vi "Read Enable and Power On Sensor Opcode_MI.vi"(8 "error in (no error)":errorcluster, 10 "Sensor name":string, 11 "MachineInterfaceRecipeOpcodes":T1) -> (0 "error out":errorcluster, 3 "Enable and Power On Sensor Opcodes":string[](array[string]))   [LabVIEW 2019, in "Machine Interface.lvclass"]
uses:
  Machine Interface.lvclass
  Controls/Machine Interface Config File Structure_MI.ctl
panel:
  out "variant":variant
  out "Error Message":string
  out "basePath in":string="$.MachineInterfaceRecipeOpcodes.TriggerLightCameraSequence[Name="
  out "output array":string[](array[string])
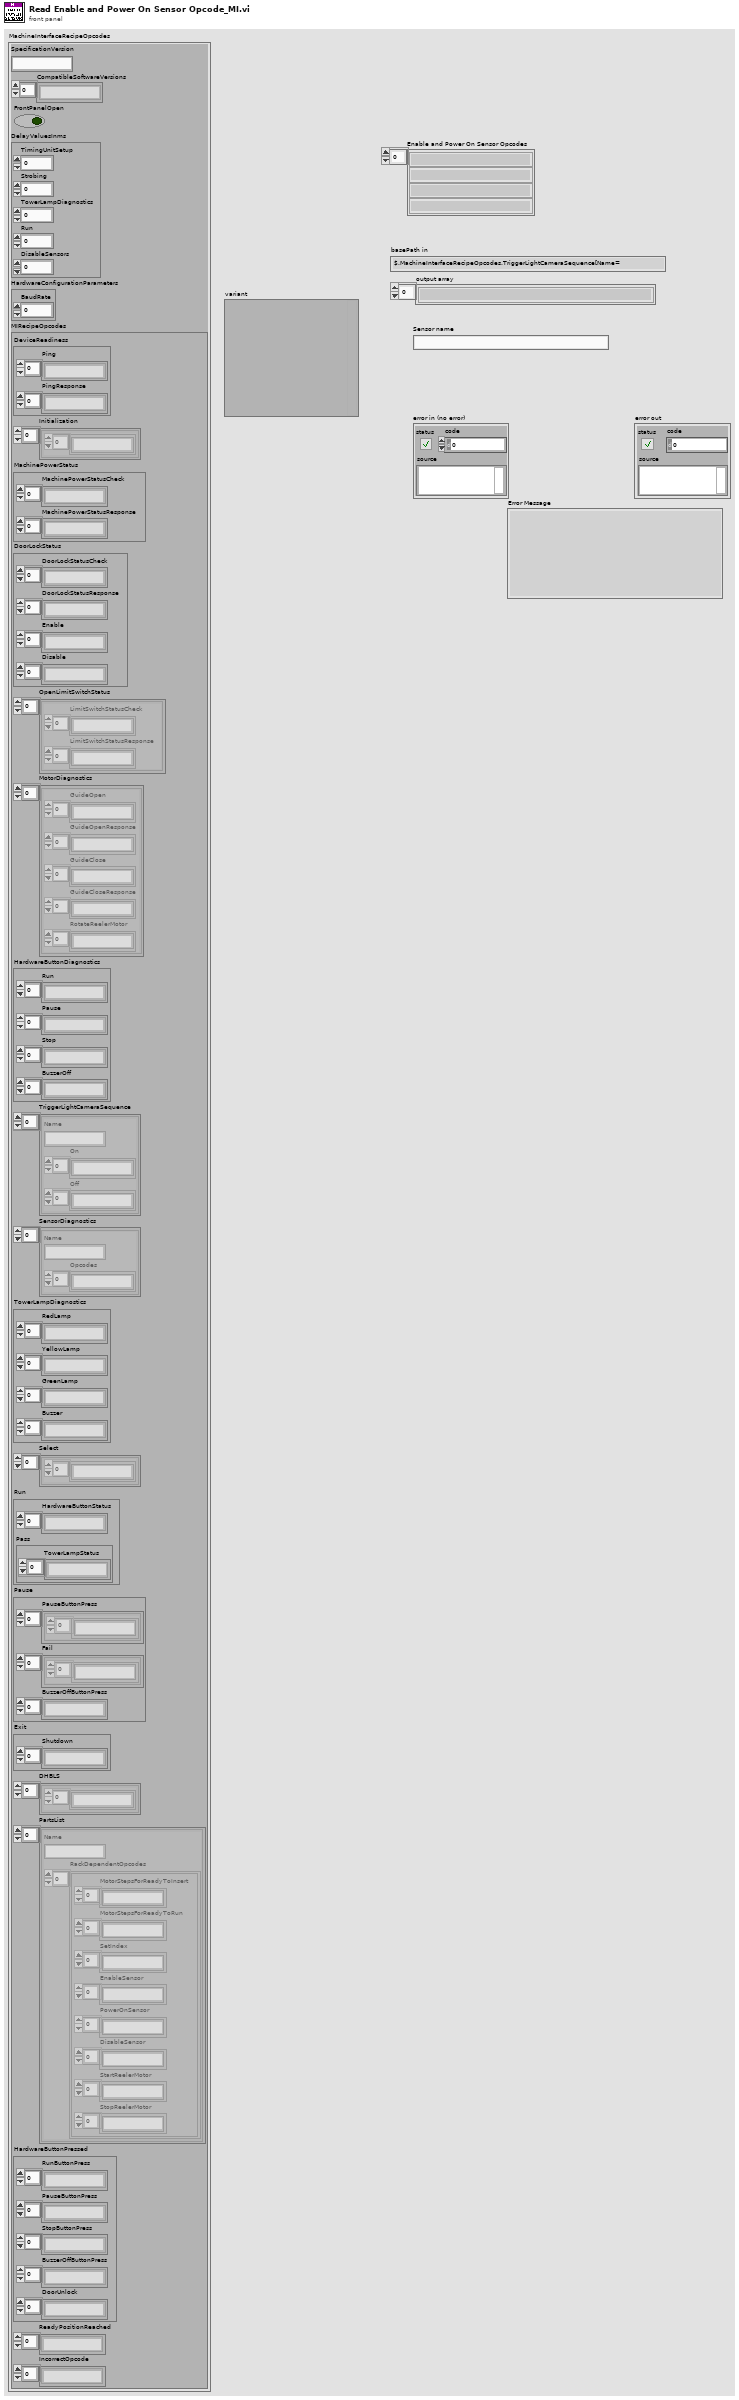
[diagram p1: front panel]
types:
  T1 = typedef "Machine Interface.lvclass/Machine Interface Config File Structure_MI.ctl" = cluster{"SpecificationVersion":string, "CompatibleSoftwareVersions":string[], "FrontPanelOpen":bool, "DelayValuesInms":cluster{"TimingUnitSetup":i32, "Strobing":i32, "TowerLampDiagnostics":i32, "Run":i32, "DisableSensors":i32}, "HardwareConfigurationParameters":cluster{"BaudRate":dbl}, "MIRecipeOpcodes":cluster{"DeviceReadiness":cluster{"Ping":string[], "PingResponse":string[]}, "Initialization":cluster{string[]}[], "MachinePowerStatus":cluster{"MachinePowerStatusCheck":string[], "MachinePowerStatusResponse":string[]}, "DoorLockStatus":cluster{"DoorLockStatusCheck":string[], "DoorLockStatusResponse":string[], "Enable":string[], "Disable":string[]}, "OpenLimitSwitchStatus":cluster{"LimitSwitchStatusCheck":string[], "LimitSwitchStatusResponse":string[]}[], "MotorDiagnostics":cluster{"GuideOpen":string[], "GuideOpenResponse":string[], "GuideClose":string[], "GuideCloseResponse":string[], "RotateReelerMotor":string[]}[], "HardwareButtonDiagnostics":cluster{"Run":string[], "Pause":string[], "Stop":string[], "BuzzerOff":string[]}, "TriggerLightCameraSequence":cluster{"Name":string, "On":string[], "Off":string[]}[], "SensorDiagnostics":cluster{"Name":string, "Opcodes":string[]}[], "TowerLampDiagnostics":cluster{"RedLamp":string[], "YellowLamp":string[], "GreenLamp":string[], "Buzzer":string[]}, "Select":cluster{string[]}[], "Run":cluster{"HardwareButtonStatus":string[], "Pass":cluster{"TowerLampStatus":string[]}}, "Pause":cluster{"PauseButtonPress":cluster{string[]}[], "Fail":cluster{string[]}[], "BuzzerOffButtonPress":string[]}, "Exit":cluster{"Shutdown":string[]}, "DHBLS":cluster{string[]}[], "PartsList":cluster{"Name":string, "RackDependentOpcodes":cluster{"MotorStepsForReadyToInsert":string[], "MotorStepsForReadyToRun":string[], "SetIndex":string[], "EnableSensor":string[], "PowerOnSensor":string[], "DisableSensor":string[], "StartReelerMotor":string[], "StopReelerMotor":string[]}[]}[], "HardwareButtonPressed":cluster{"RunButtonPress":string[], "PauseButtonPress":string[], "StopButtonPress":string[], "BuzzerOffButtonPress":string[], "DoorUnlock":string[]}, "ReadyPositionReached":string[], "IncorrectOpcode":string[]}}
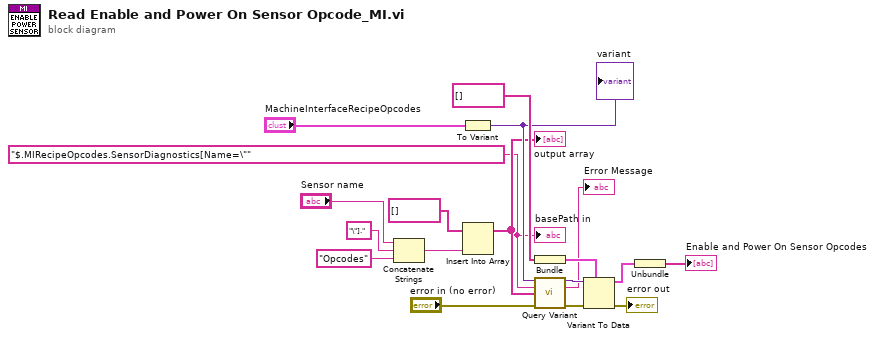
[diagram p0: block diagram]
diagram:
  w2 = "$.MIRecipeOpcodes.SensorDiagnostics[Name=\"" ("basePath in")
  n1 = Concatenate Strings("Sensor name", "\"]." ("string"), "Opcodes" ("string")) -> (w17:string)
  n2 = To Variant(anything="MachineInterfaceRecipeOpcodes") -> (Variant=w7:variant)
  "variant" <- w7
  n3 = Insert Into Array(array=string[] [] ("Array"), new element=w17) -> (w3:string[])  [unwired: 1 in]
  "output array" <- w3
  n4 = Bundle(string[] []) -> (w14:cluster{string[]})  [unwired: 1 in]
  n5 = call <vilib>:"Query Variant.vi"("VCluster in"=w7, "basePath in"=w2, "pathList"=w3, "error IO"="error in (no error)") -> ("VCluster\n out"=w6:variant, "Error Message"=→"Error Message":string, "error out"=w4:errorcluster)  [unwired: 8 in, 1 out]
  n6 = Variant To Data(error in=w4, type=w14, Variant=w6) -> (data=w15:cluster{string[]}, error out=→"error out":errorcluster)
  n7 = Unbundle(w15) -> (→"Enable and Power On Sensor Opcodes":string[])
  "basePath in" <- w2
